vi "获取采配水运行状态.vi"(8 "error in (no error)":errorcluster) -> (0 "error out":errorcluster, 3 "运行流程":T1)   [LabVIEW 2016, in "质控单元V1.lvlib"]
uses:
  <vilib>/Plasmionique/MB Master/MB Master.lvlib
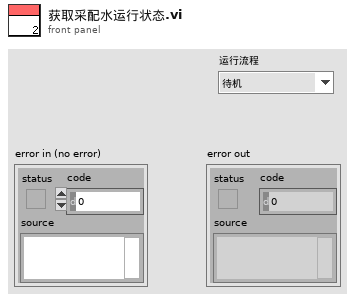
[diagram p1: front panel]
types:
  T1 = typedef "质控单元V1.lvlib/采配水通用流程.ctl" = enum16{"待机", "润洗", "采样", "沉淀", "配水", "反冲洗", "结束"}
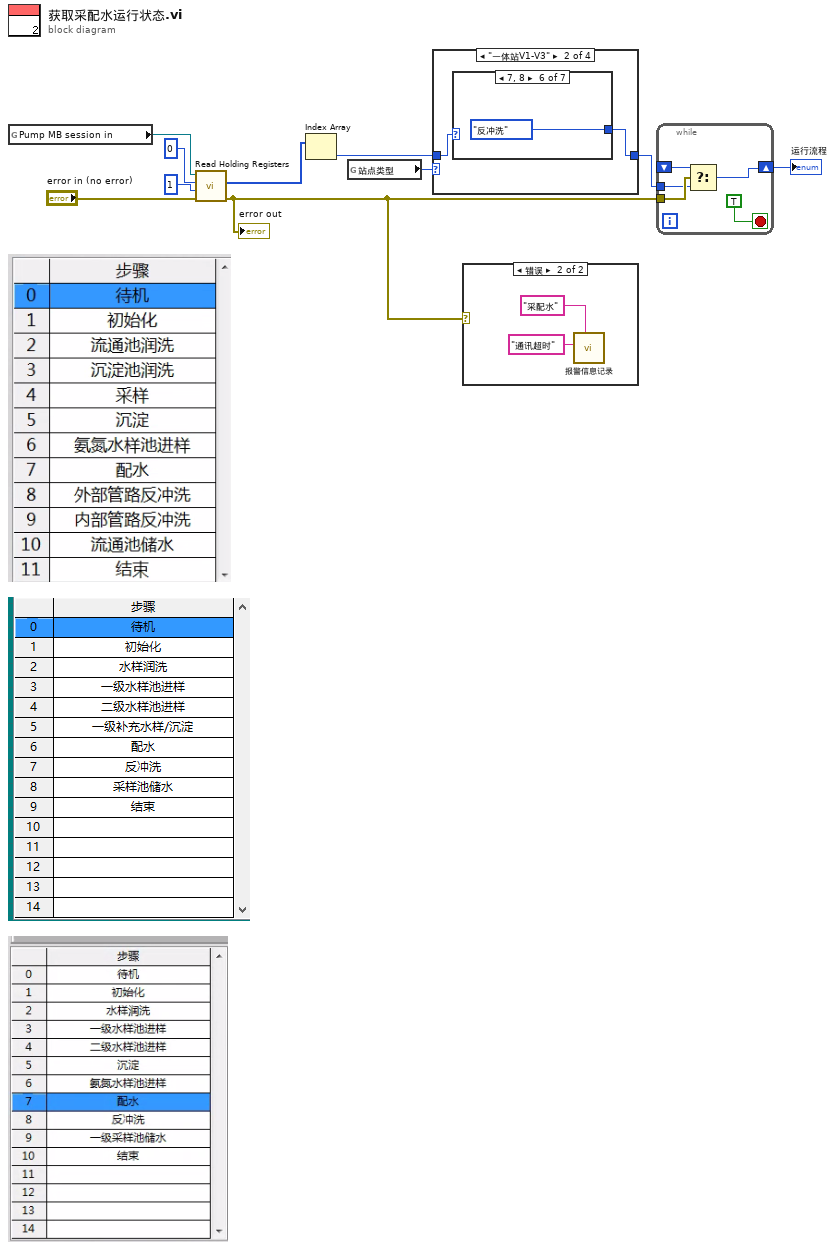
[diagram p0: block diagram]
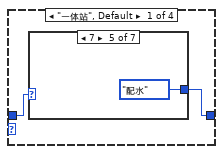
[diagram p3: hidden frame]
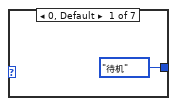
[diagram p4: hidden frame]
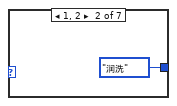
[diagram p5: hidden frame]
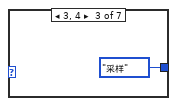
[diagram p6: hidden frame]
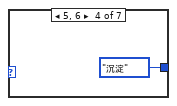
[diagram p7: hidden frame]
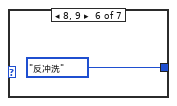
[diagram p8: hidden frame]
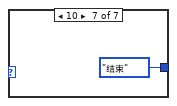
[diagram p9: hidden frame]
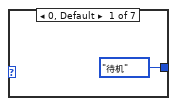
[diagram p10: hidden frame]
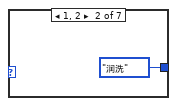
[diagram p11: hidden frame]
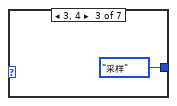
[diagram p12: hidden frame]
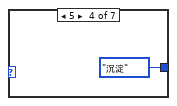
[diagram p13: hidden frame]
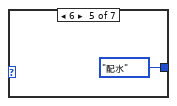
[diagram p14: hidden frame]
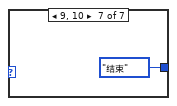
[diagram p15: hidden frame]
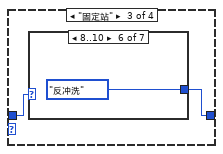
[diagram p16: hidden frame]
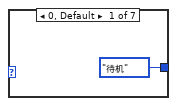
[diagram p17: hidden frame]
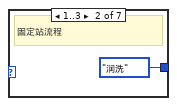
[diagram p18: hidden frame]
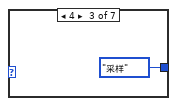
[diagram p19: hidden frame]
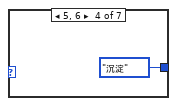
[diagram p20: hidden frame]
diagram:
  n1 = global read "系统交互.vi" "Pump MB session in"() -> (w9:refnum<class "MB_Master.lvclass">)
  n2 = call <vilib>:"Read Holding Registers.vi"("error in (no error)"="error in (no error)", "quantity"=u16 1, "starting address"=u16 0, "MB session in"=w9) -> ("error out"=w1:errorcluster, "Registers"=w6:u16[])  [unwired: 5 in, 1 out]
  "error out" <- w1
  n3 = Index Array(array=w6) -> (element=w5:u16)  [unwired: 1 in]
  n4 = global read "系统交互.vi" "站点类型"() -> (w4:enum16{"一体站", "固定站", "浮船", "一体站V1-V3"})
  n5 = case shown="\"一体站V1-V3\"" w4 {
    tunnel: [w12 w21 w30 w38] -> w3
    tunnel: w5 -> [w11 w20 w29 w38]
    frame "一体站", Default {
      n6 = case shown="7" w11 {
        tunnel: [采配水通用流程."待机" ("运行流程 2") 采配水通用流程."润洗" ("运行流程 2") 采配水通用流程."采样" ("运行流程 2") 采配水通用流程."沉淀" ("运行流程 2") 采配水通用流程."配水" ("运行流程 2") 采配水通用流程."反冲洗" ("运行流程 2") 采配水通用流程."结束" ("运行流程 2")] -> w12
        frame 0, Default {
        }
        frame 1, 2 {
        }
        frame 3, 4 {
        }
        frame 5, 6 {
        }
        frame 7 {
        }
        frame 8, 9 {
        }
        frame 10 {
        }
      }
    }
    frame "一体站V1-V3" {
      n7 = case shown="7, 8" w20 {
        tunnel: [采配水通用流程."待机" ("运行流程 2") 采配水通用流程."润洗" ("运行流程 2") 采配水通用流程."采样" ("运行流程 2") 采配水通用流程."沉淀" ("运行流程 2") 采配水通用流程."配水" ("运行流程 2") 采配水通用流程."反冲洗" ("运行流程 2") 采配水通用流程."结束" ("运行流程 2")] -> w21
        frame 0, Default {
        }
        frame 1, 2 {
        }
        frame 3, 4 {
        }
        frame 5 {
        }
        frame 6 {
        }
        frame 7, 8 {
        }
        frame 9, 10 {
        }
      }
    }
    frame "固定站" {
      n8 = case shown="8..10" w29 {
        tunnel: [采配水通用流程."待机" ("运行流程 2") 采配水通用流程."润洗" ("运行流程 2") 采配水通用流程."采样" ("运行流程 2") 采配水通用流程."沉淀" ("运行流程 2") 采配水通用流程."配水" ("运行流程 2") 采配水通用流程."反冲洗" ("运行流程 2") 采配水通用流程."结束" ("运行流程")] -> w30
        frame 0, Default {
        }
        frame 1..3 {
          # "固定站流程"
        }
        frame 4 {
        }
        frame 5, 6 {
        }
        frame 7 {
        }
        frame 8..10 {
        }
        frame 11 {
        }
      }
    }
    frame "浮船" {
    }
  }
  n9 = case shown="错误" w1 {
    frame No Error {
    }
    frame Error {
      n10 = call "报警信息记录.vi"("参数"="采配水", "报警信息"="通讯超时") -> ()  [unwired: 9 in, 1 out]
    }
  }
  n11 = while {
    shift-right: [w41] -> w2
    shift-left: _ -> [w43]
    tunnel: w3 -> [w42]
    tunnel: w1 -> [w44]
    stop <- TRUE stop-if-true
    n12 = Select(t=w43, s=w44, f=w42) -> (s? t:f=w41:u16)
  }
  "运行流程" <- w2
